vi "Get I32Array.vi"(8 "error in (no error)":errorcluster, 11 "I32ArrayMsg in":refnum<class "I32ArrayMsg.lvclass">) -> (0 "error out":errorcluster, 2 "Message Data":i32[](array[numeric]), 3 "I32ArrayMsg out":refnum<class "I32ArrayMsg.lvclass">)   [LabVIEW 2009, in "LapDog.Messaging.v2.NativeArrays.lvlib" / "I32ArrayMsg.lvclass"]
doc: "Returns the data contained in the message.\n\nThis method executes regardless of the error in state."
uses:
  I32ArrayMsg.lvclass
  I32ArrayMsg.lvclass/I32ArrayMsg.ctl
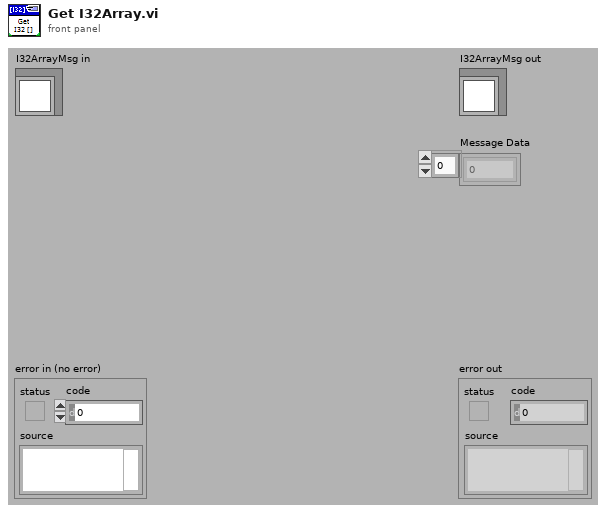
[diagram p1: front panel]
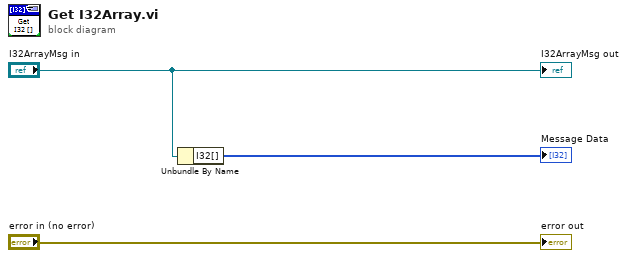
[diagram p0: block diagram]
diagram:
  n1 = Unbundle By Name("I32ArrayMsg in") -> ("I32[]"=→"Message Data":i32[])
  "error out" <- "error in (no error)"
  "I32ArrayMsg out" <- "I32ArrayMsg in"
